vi "Main.vi"() -> ()   [LabVIEW 2019]
uses:
  main_control.ctl
  invader.ctl
  <vilib>/picture/picture.llb/imagedata.ctl
  move_dir_lr.ctl
  <vilib>/Utility/miscctls.llb/LVBoundsTypeDef.ctl
  shot_direction.ctl
  <vilib>/numeric/Random Number (Range) U64.vi
  <vilib>/numeric/Random Number (Range) DBL.vi
  <vilib>/numeric/sub_Random U32.vi
  <vilib>/Utility/inputDevices.llb/keyboardAcquire.vi
panel:
  out "output cluster":cluster{"x":i16, "y":i16}
  out "ShotPos_OUT":T1(array[cluster])
  in  "shotwidth":i16=10
  in  "speed":i16=10
  in  "smoothness":u32=10
  out "game":picture
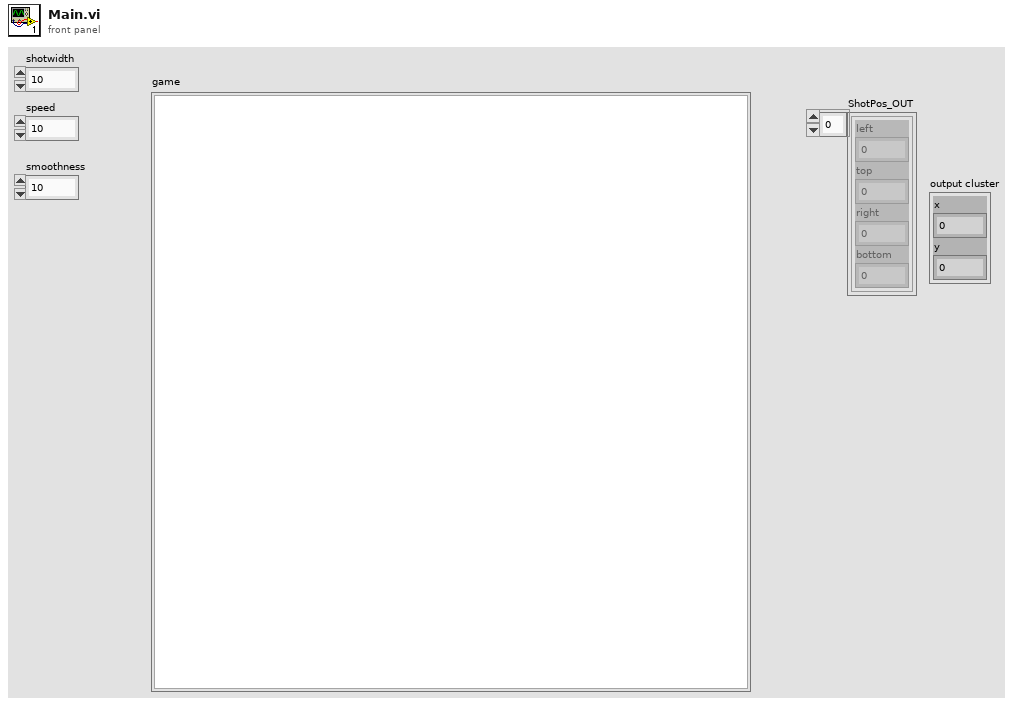
[diagram p1: front panel]
types:
  T1 = cluster{"left":i16, "top":i16, "right":i16, "bottom":i16}[]
  T2 = cluster{"left":i16, "top":i16, "right":i16, "bottom":i16}
  T3 = typedef "move_dir_lr.ctl" = enum16{"right", "left"}
  T4 = typedef "invader.ctl" = cluster{"output cluster":T5, "direction":T3, "shot_period":dbl, "Speed":i16, "Bounds":T6}
  T5 = typedef "imagedata.ctl" = cluster{"image type":i32, "image depth":i32, "image":u8[], "mask":u8[], "colors":u32[], "Rectangle":cluster{"left":i16, "top":i16, "right":i16, "bottom":i16}}
  T6 = typedef "LVBoundsTypeDef.ctl" = cluster{"Width":u32, "Height":u32}
  T7 = typedef "main_control.ctl" = enum16{"Idle", "RedrawPic"}
  T8 = typedef "shot_direction.ctl" = enum16{"down", "up"}
  T9 = cluster{"Font Name:":string, "Size":i16, "Strikeout?":bool, "Italic?":bool, "Underline?":bool, "Outline?":bool, "Shadow?":bool, "Bold?":bool}
  T10 = enum16{"User-specified Font", "Application Font", "System Font", "Dialog Font"}
  T11 = enum16{"0", "1", "2", "3", "4", "5", "6", "7", "8", "9", "A", "B", "C", "D", "E", "F", "G", "H", "I", "J", "K", "L", "M", "N", "O", "P", "Q", "R", "S", "T", "U", "V", "W", "X", "Y", "Z", "F1", "F2", "F3", "F4", "F5", "F6", "F7", "F8", "F9", "F10", "F11", "F12", "F13", "F14", "F15", "ADD", "BACK", "BACKSLASH", "CAPITAL", "COMMA", "DECIMAL", "DELETE", "DIVIDE", "DOWN", "END", "EQUALS", "ESCAPE", "GRAVE (`)", "HOME", "INSERT", "LBRACKET", "LCONTROL", "LEFT", "L ALT", "LSHIFT", "LWIN", "MINUS", "MULTIPLY", "NEXT", "NUMLOCK", "NUMPAD_0", "NUMPAD_1", "NUMPAD_2", "NUMPAD_3", "NUMPAD_4", "NUMPAD_5", "NUMPAD_6", "NUMPAD_7", "NUMPAD_8", "NUMPAD_9", "PAUSE", "PERIOD", "PRIOR (PG UP)", "RBRACKET", "RCONTROL", "RETURN", "RIGHT", "R ALT", "RSHIFT", "RWIN", "SCROLL", "SEMICOLON", "SLASH", "SPACE", "SUBTRACT", "TAB", "UP", "ENTER (num pad)", "' (quote)"}[]
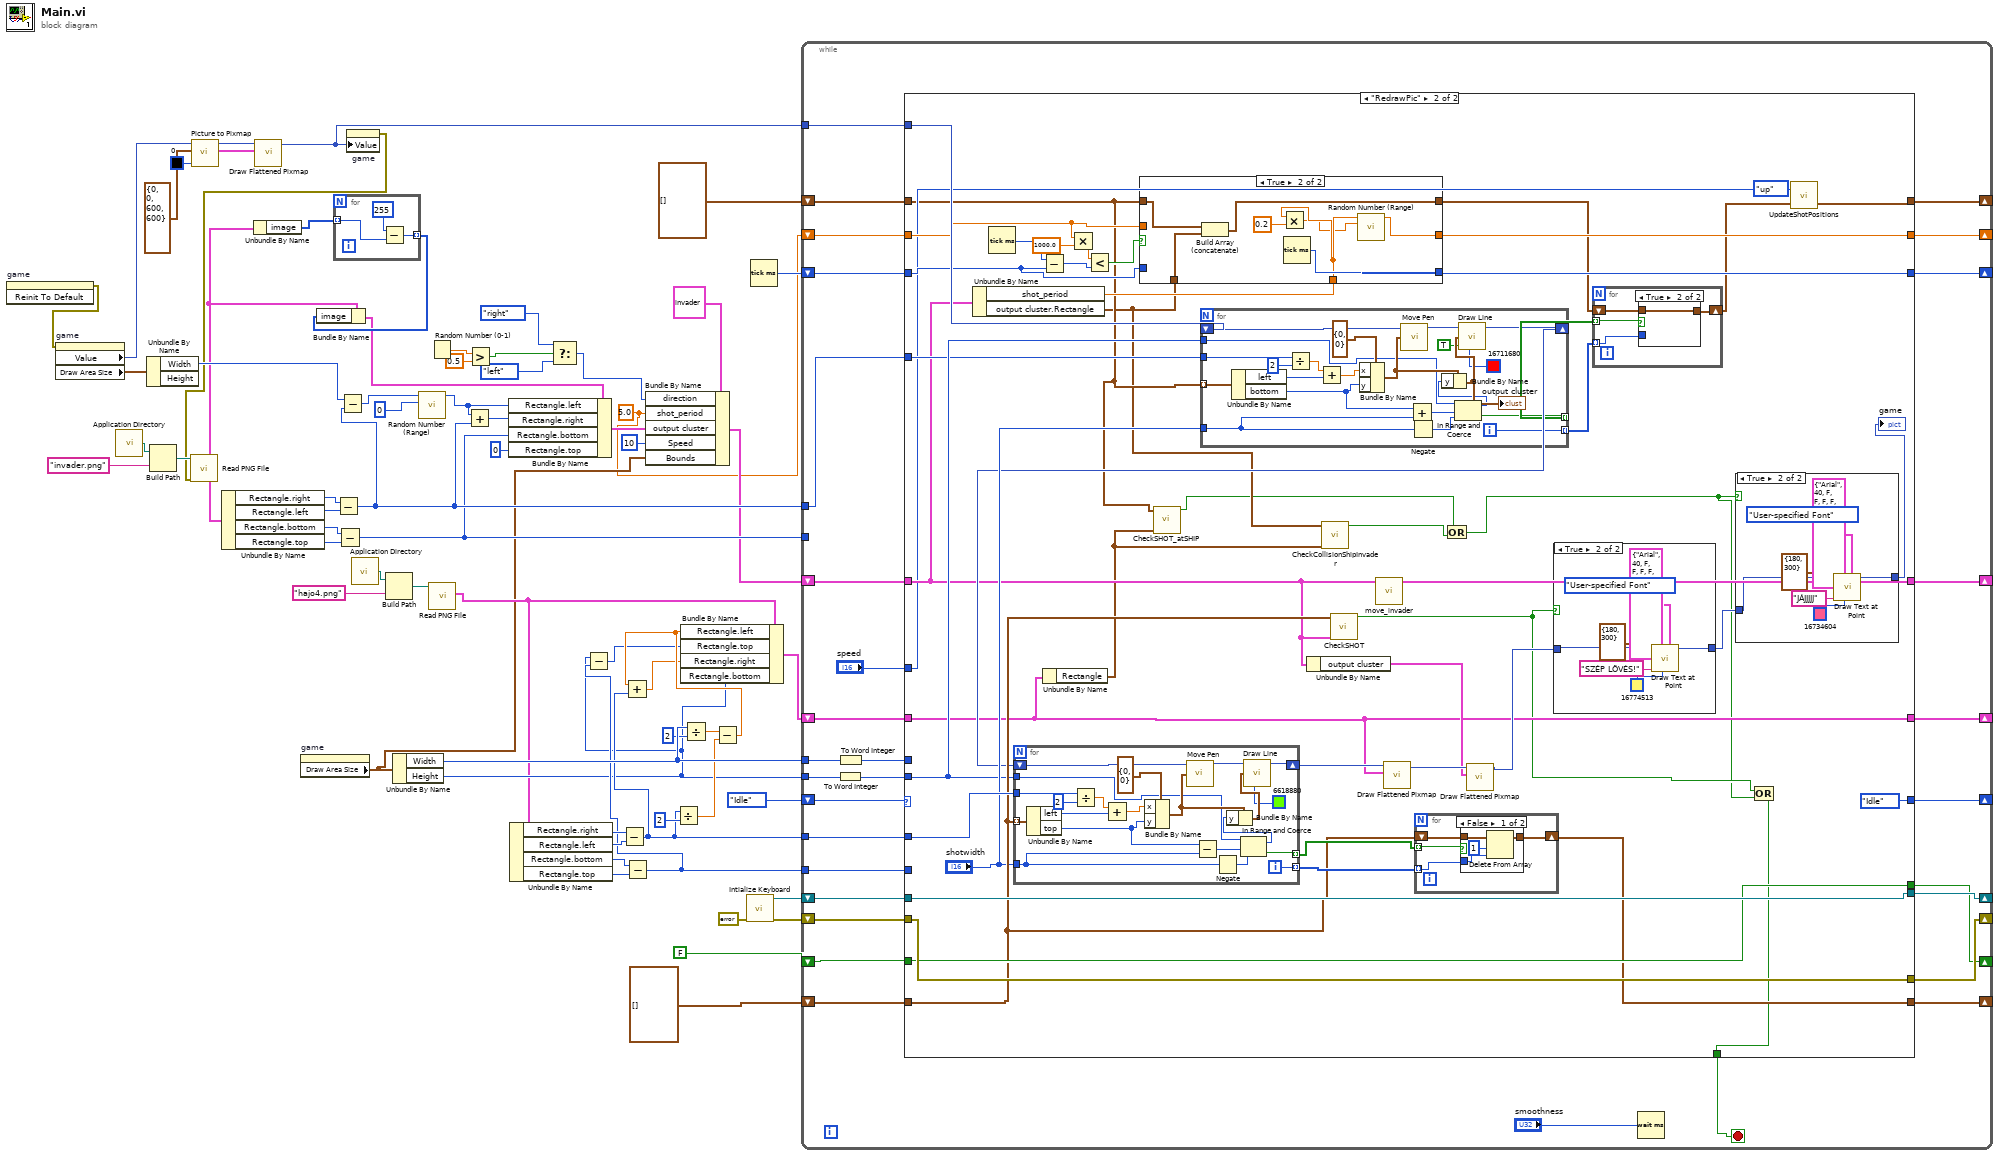
[diagram p0: block diagram]
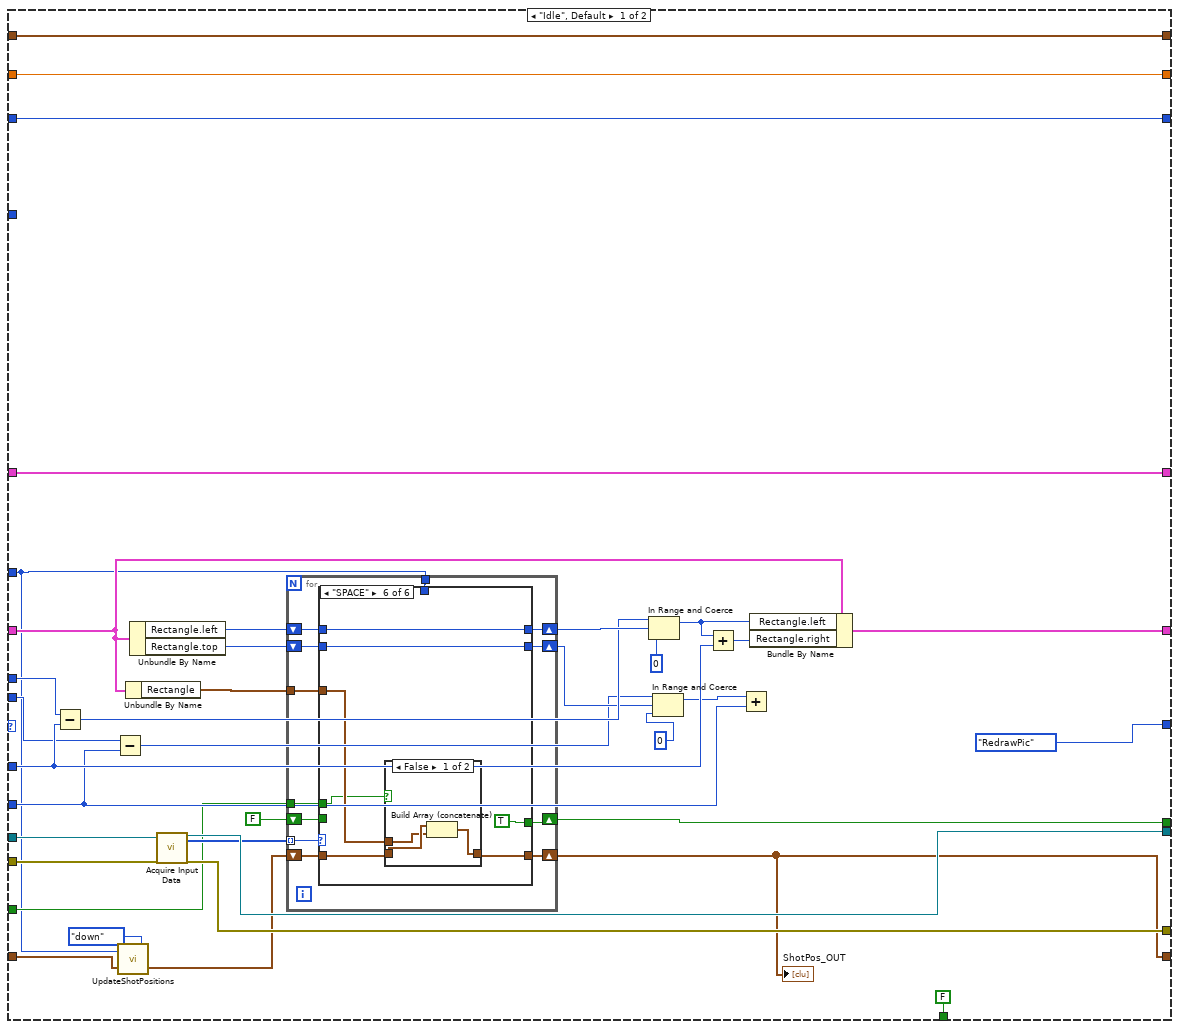
[diagram p2: hidden frame]
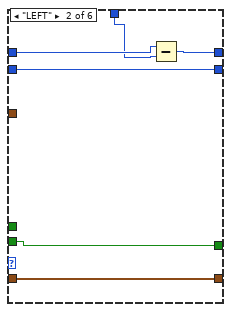
[diagram p4: hidden frame]
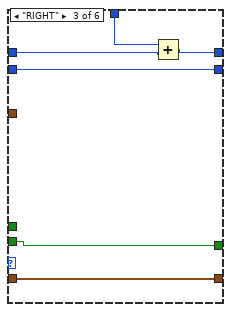
[diagram p5: hidden frame]
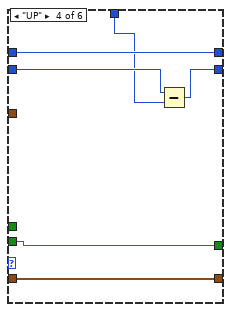
[diagram p6: hidden frame]
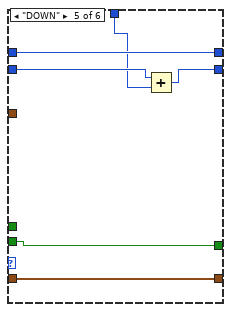
[diagram p7: hidden frame]
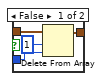
[diagram p10: hidden frame]
diagram:
  w1 = 5.0 ("shot_period")
  n1 = invoke on="game" class="Pict" method="Reinit To Default"() -> (error out=w4:errorcluster)  [unwired: 3 in, 2 out]
  n2 = property on="game" class="Pict"(error in=w4) -> ("Value"=w11:picture, "Draw Area Size"=w35:T6)  [unwired: 1 in, 2 out]
  n3 = call <vilib>:"Application Directory.vi"() -> ("Application Directory"=w41:path)
  n4 = Unbundle By Name(w35) -> ("Width"=w34:u32)  [unwired: 1 out]
  n5 = Build Path(base path=w41, name or relative path="invader.png") -> (appended path=w43:path)
  n6 = call <vilib>:"Picture to Pixmap.vi"("Background Color"=u32 0, "rect"=T2 {"left"=0, "top"=0, "right"=600, "bottom"=600}, "picture"=w11) -> ("image data"=w7:T5, "new picture"=w8:picture)  [unwired: 7 in]
  n7 = call <vilib>:"Draw Flattened Pixmap.vi"("image data"=w7, "picture"=w8) -> ("new picture"=w5:picture)  [unwired: 7 in]
  n8 = property on="game" class="Pict"() -> ("Draw Area Size"=w16:T6)  [unwired: 2 in, 2 out]
  n9 = property on="game" class="Pict"("Value"=w5) -> (error out=w6:errorcluster)  [unwired: 2 in, 1 out]
  n10 = call <vilib>:"Read PNG File.vi"("error in (no error)"=w6, "path to PNG file"=w43) -> ("image data"=w14:T5)  [unwired: 7 in, 2 out]
  n11 = Unbundle By Name(w14) -> ("Rectangle.right"=w40:i16, "Rectangle.left"=w39:i16, "Rectangle.bottom"=w38:i16, "Rectangle.top"=w37:i16)
  n12 = Unbundle By Name(w14) -> ("image"=w15:u8[])
  n13 = for {
    tunnel: w15 -> [w70] mode=indexing
    tunnel: [w69] -> w13 mode=indexing
    n14 = Subtract(x=u8 255, y=w70) -> (x-y=w69:u8)
  }
  n15 = Bundle By Name(cluster=w14, "image"=w13) -> (w12:T5)
  n16 = Subtract(x=w40, y=w39) -> (x-y=w31:i16)
  n17 = Subtract(x=w38, y=w37) -> (x-y=w28:i16)
  n18 = Subtract(x=w34, y=w31) -> (x-y=w33:u32)
  n19 = call <vilib>:"Application Directory.vi"() -> ("Application Directory"=w68:path)
  n20 = Build Path(base path=w68, name or relative path="hajo4.png") -> (appended path=w66:path)
  n21 = Unbundle By Name(w16) -> ("Width"=w55:u32, "Height"=w45:u32)
  n22 = call-poly <vilib>:"Random Number (Range).vi"("lower bound (0)"=u64 0, "upper bound (100)"=w33) -> ("number"=w32:u64)  [unwired: 9 in]
  n23 = Random Number (0-1)() -> (number: 0 to 1=w24:dbl)
  n24 = call <vilib>:"Read PNG File.vi"("path to PNG file"=w66) -> ("image data"=w18:T5)  [unwired: 8 in, 2 out]
  n25 = Add(x=w32, y=w31) -> (x+y=w30:u64)
  n26 = Greater?(x=w24, y=0.5) -> (0:w22:bool)
  n27 = Bundle By Name(cluster=w12, "Rectangle.left"=w32, "Rectangle.right"=w30, "Rectangle.bottom"=w28, "Rectangle.top"=i16 0) -> (w25:T5)
  n28 = Unbundle By Name(w18) -> ("Rectangle.right"=w65:i16, "Rectangle.left"=w64:i16, "Rectangle.bottom"=w63:i16, "Rectangle.top"=w62:i16)
  n29 = Select(t=move_dir_lr."right" ("direction"), s=w22, f=move_dir_lr."left" ("direction")) -> (s? t:f=w19:T3)
  n30 = Subtract(x=w65, y=w64) -> (x-y=w49:i16)
  n31 = Subtract(x=w63, y=w62) -> (x-y=w47:i16)
  n32 = Subtract(x=w45, y=w47) -> (x-y=w46:u32)
  n33 = Bundle By Name(cluster=T4 {"output cluster"={"image type"=0, "image depth"=0, "image"=[], "mask"=[], "colors"=[], "Rectangle"={"left"=0, "top"=0, "right"=0, "bottom"=0}}, "direction"=enum."right", "shot_period"=0.0, "Speed"=10, "Bounds"={"Width"=0, "Height"=0}} ("input cluster"), "direction"=w19, "shot_period"=w1, "output cluster"=w25, "Speed"=i16 10, "Bounds"=w16) -> (w26:T4)
  n34 = Divide(x=w49, y=u32 2) -> (x/y=w51:dbl)
  n35 = Divide(x=w55, y=u32 2) -> (x/y=w53:dbl)
  n36 = Subtract(x=w53, y=w51) -> (x-y=w50:dbl)
  n37 = Add(x=w50, y=w49) -> (x+y=w48:dbl)
  n38 = Bundle By Name(cluster=w18, "Rectangle.left"=w50, "Rectangle.top"=w46, "Rectangle.right"=w48, "Rectangle.bottom"=w45) -> (w44:T5)
  n39 = call <vilib>:"Intialize Keyboard.vi"("error in (no error)"=errorcluster {"status"=FALSE, "code"=0, "source"=""}) -> ("error out"=w59:errorcluster, "device ID"=w60:refnum<k1>)  [unwired: 9 in]
  n40 = Tick Count (ms)() -> (millisecond timer value=w2:u32)
  n41 = while {
    tunnel: w49 -> [w102]
    tunnel: w55 -> [w93]
    tunnel: w47 -> [w99]
    tunnel: w45 -> [w88]
    shift-right: [w96] -> _
    shift-left: main_control."Idle" -> [w98]
    shift-right: [w97] -> _
    shift-left: w44 -> [w101]
    shift-right: [w90] -> _
    shift-left: w60 -> [w95]
    shift-right: [w89] -> _
    shift-left: w59 -> [w94]
    shift-right: [w85] -> _
    shift-left: T1 [] -> [w86]
    shift-right: [w83] -> _
    shift-left: FALSE -> [w84]
    tunnel: w31 -> [w76]
    tunnel: w28 -> [_]
    shift-right: [w81] -> _
    shift-left: w26 -> [w82]
    tunnel: w5 -> [w80]
    shift-right: [w78] -> _
    shift-left: T1 [] -> [w79]
    shift-right: [w75] -> _
    shift-left: w2 -> [w77]
    shift-right: [w73] -> _
    shift-left: w1 -> [w74]
    stop <- w91 stop-if-true
    n42 = To Word Integer(number=w88) -> (16bit integer=w87:i16)
    n43 = To Word Integer(number=w93) -> (16bit integer=w92:i16)
    n44 = case shown="\"RedrawPic\"" w98 {
      tunnel: w101 -> [w118 w200]
      tunnel: [w135 w200] -> w97
      tunnel: [main_control."RedrawPic" main_control."Idle"] -> w96
      tunnel: w102 -> [w136 w234]
      tunnel: w99 -> [w120 _]
      tunnel: w92 -> [w137 _]
      tunnel: w87 -> [w125 w222]
      tunnel: w95 -> [w139 w237]
      tunnel: w94 -> [w138 w236]
      tunnel: [FALSE ("SHOT") w196] -> w91
      tunnel: [w134 w237] -> w90
      tunnel: [w133 w236] -> w89
      tunnel: w86 -> [w114 w226]
      tunnel: [w115 w227] -> w85
      tunnel: w84 -> [w112 w231]
      tunnel: [w110 w231] -> w83
      tunnel: w82 -> [w109 w220]
      tunnel: [w109 w228] -> w81
      tunnel: w80 -> [_ w224]
      tunnel: w79 -> [w107 w201]
      tunnel: [w107 w204] -> w78
      tunnel: w77 -> [w105 w215]
      tunnel: w76 -> [_ w221]
      tunnel: [w105 w216] -> w75
      tunnel: w74 -> [w106 w209]
      tunnel: [w106 w214] -> w73
      tunnel: "speed" -> [w104 w206]
      frame "Idle", Default {
        n45 = Subtract(x=w137, y=w136) -> (x-y=w128:i16)
        n46 = Subtract(x=w125, y=w120) -> (x-y=w121:i16)
        n47 = call "UpdateShotPositions.vi"("Direction"=shot_direction."down", "ShotPos_IN"=w114, "Speed"=w104) -> ("ShotPos_OUT"=w116:T1)
        n48 = Unbundle By Name(w118) -> ("Rectangle"=w117:T2)
        n49 = Unbundle By Name(w118) -> ("Rectangle.left"=w131:i16, "Rectangle.top"=w124:i16)
        n50 = call-poly <vilib>:"Acquire Input Data.vi"("device ID"=w139, "error in (no error)"=w138) -> ("device ID"=w134:refnum<k1>, "keys pressed"=w132:T11, "error out"=w133:errorcluster)  [unwired: 15 in]
        n51 = for {
          tunnel: w132 -> [w151] mode=indexing
          shift-right: [w150] -> w130
          shift-left: w131 -> [w149]
          shift-right: [w147] -> w122
          shift-left: w124 -> [w148]
          tunnel: w104 -> [w146]
          tunnel: w117 -> [w145]
          shift-right: [w143] -> w115
          shift-left: w116 -> [w144]
          shift-right: [w141] -> w110
          shift-left: FALSE -> [w142]
          tunnel: w112 -> [w140]
          n52 = case shown="\"SPACE\"" w151 {
            tunnel: w149 -> [w155 w160 w166 w173 w179 w186]
            tunnel: [w155 w158 w165 w173 w179 w186] -> w150
            tunnel: w148 -> [w154 w161 w167 w172 w178 w185]
            tunnel: [w154 w161 w167 w170 w176 w185] -> w147
            tunnel: w146 -> [_ w159 w164 w171 w177 _]
            tunnel: w145 -> [_ _ _ _ _ w183]
            tunnel: w144 -> [w153 w157 w163 w169 w175 w184]
            tunnel: [w153 w157 w163 w169 w175 w182] -> w143
            tunnel: w142 -> [w152 w156 w162 w168 w174 _]
            tunnel: [w152 w156 w162 w168 w174 TRUE] -> w141
            tunnel: w140 -> [_ _ _ _ _ w181]
            frame Default {
            }
            frame "LEFT" {
              n53 = Subtract(x=w160, y=w159) -> (x-y=w158:i16)
            }
            frame "RIGHT" {
              n54 = Add(x=w164, y=w166) -> (x+y=w165:i16)
            }
            frame "UP" {
              n55 = Subtract(x=w172, y=w171) -> (x-y=w170:i16)
            }
            frame "DOWN" {
              n56 = Add(x=w178, y=w177) -> (x+y=w176:i16)
            }
            frame "SPACE" {
              n57 = case shown="False" w181 {
                tunnel: w184 -> [w189 w190]
                tunnel: w183 -> [w188 _]
                tunnel: [w187 w190] -> w182
                frame False {
                  n58 = Build Array (concatenate)(w189, w188) -> (w187:T1)
                }
                frame True {
                }
              }
            }
          }
        }
        "ShotPos_OUT" <- w115
        n59 = In Range and Coerce(upper limit=w128, x=w130, lower limit=i16 0) -> (coerced(x)=w127:i16)  [unwired: 1 out]
        n60 = In Range and Coerce(upper limit=w121, x=w122, lower limit=i16 0) -> (coerced(x)=w119:i16)  [unwired: 1 out]
        n61 = Add(x=w127, y=w136) -> (x+y=w126:i16)
        n62 = Add(x=w119, y=w120) -> ()  [unwired: 1 out]
        n63 = Bundle By Name(cluster=w118, "Rectangle.left"=w127, "Rectangle.right"=w126) -> (w135:T5)
      }
      frame "RedrawPic" {
        n64 = Unbundle By Name(w220) -> ("shot_period"=w213:dbl, "output cluster.Rectangle"=w195:T2)
        n65 = Tick Count (ms)() -> (millisecond timer value=w219:u32)
        n66 = Subtract(x=w219, y=w215) -> (x-y=w218:u32)
        n67 = Unbundle By Name(w200) -> ("Rectangle"=w194:T2)
        n68 = Multiply(x=w209, y=1000.0) -> (x*y=w207:dbl)
        n69 = Less?(x=w207, y=w218) -> (x < y?=w217:bool)
        n70 = case shown="True" w217 {
          tunnel: w201 -> [w258 w266]
          tunnel: w195 -> [_ w265]
          tunnel: [w258 w264] -> w210
          tunnel: [w257 w263] -> w216
          tunnel: w215 -> [w257 _]
          tunnel: [w256 w259] -> w214
          tunnel: w213 -> [_ w262]
          tunnel: w209 -> [w256 _]
          frame False {
          }
          frame True {
            n71 = Build Array (concatenate)(w266, w265) -> (w264:T1)
            n72 = Multiply(x=w262, y=0.2) -> (x*y=w260:dbl)
            n73 = Tick Count (ms)() -> (millisecond timer value=w263:u32)
            n74 = call-poly <vilib>:"Random Number (Range).vi"("lower bound (0)"=w260, "upper bound (100)"=w262) -> ("number"=w259:dbl)  [unwired: 9 in]
          }
        }
        n75 = call "CheckSHOT_atSHIP.vi"("ShipRectangle"=w194, "InvaderShotArray"=w201) -> ("SHOT"=w192:bool)  [unwired: 9 in]
        n76 = for {
          tunnel: w201 -> [w287] mode=indexing
          shift-right: [w275] -> w223
          shift-left: w224 -> [w288]
          tunnel: w221 -> [w286]
          tunnel: [w274] -> w212 mode=indexing
          tunnel: w222 -> [w268]
          tunnel: [w271] -> w211 mode=indexing
          tunnel: "shotwidth" -> [w269]
          i -> [w271]
          n77 = Unbundle By Name(w287) -> ("left"=w283:i16, "bottom"=w278:i16)
          n78 = Divide(x=w286, y=i16 2) -> (x/y=w284:dbl)
          n79 = Add(x=w284, y=w283) -> (x+y=w282:dbl)
          n80 = Bundle By Name(cluster=cluster{"x":i16, "y":i16} {"x"=0, "y"=0} ("new position"), "x"=w282, "y"=w278) -> (w279:cluster{"x":i16, "y":i16})
          n81 = call <vilib>:"Move Pen.vi"("new position"=w279, "picture"=w288) -> ("new picture"=w281:picture)  [unwired: 3 in]
          n82 = Add(x=w278, y=w269) -> (x+y=w273:i16)
          n83 = Negate(x=w269) -> (-x=w267:i16)
          n84 = In Range and Coerce(upper limit=w268, x=w273, lower limit=w267) -> (coerced(x)=w272:i16, In Range?=w274:bool)
          n85 = Bundle By Name(cluster=w279, "y"=w272) -> (w277:cluster{"x":i16, "y":i16})
          "output cluster" <- w277
          n86 = call <vilib>:"Draw Line.vi"("picture"=w281, "end point"=w277, "absolute coordinates?(T)"=TRUE, "color(black)"=u32 16711680) -> ("new picture"=w275:picture)  [unwired: 5 in]
        }
        n87 = for {
          tunnel: w226 -> [w325] mode=indexing
          shift-right: [w314] -> w235
          shift-left: w223 -> [w326]
          tunnel: w234 -> [w324]
          tunnel: [w313] -> w232 mode=indexing
          tunnel: w222 -> [w310]
          tunnel: [w308] -> w233 mode=indexing
          tunnel: "shotwidth" -> [w306]
          i -> [w308]
          n88 = Unbundle By Name(w325) -> ("left"=w321:i16, "top"=w316:i16)
          n89 = Divide(x=w324, y=i16 2) -> (x/y=w322:dbl)
          n90 = Add(x=w322, y=w321) -> (x+y=w320:dbl)
          n91 = Bundle By Name(cluster=cluster{"x":i16, "y":i16} {"x"=0, "y"=0} ("new position"), "x"=w320, "y"=w316) -> (w317:cluster{"x":i16, "y":i16})
          n92 = call <vilib>:"Move Pen.vi"("new position"=w317, "picture"=w326) -> ("new picture"=w319:picture)  [unwired: 3 in]
          n93 = Subtract(x=w316, y=w306) -> (x-y=w312:i16)
          n94 = Negate(x=w306) -> (-x=w311:i16)
          n95 = In Range and Coerce(upper limit=w310, x=w312, lower limit=w311) -> (coerced(x)=w309:i16, In Range?=w313:bool)
          n96 = Bundle By Name(cluster=w317, "y"=w309) -> (w315:cluster{"x":i16, "y":i16})
          n97 = call <vilib>:"Draw Line.vi"("picture"=w319, "end point"=w315, "color(black)"=u32 6618880) -> ("new picture"=w314:picture)  [unwired: 6 in]
        }
        n98 = Unbundle By Name(w220) -> ("output cluster"=w229:T5)
        n99 = call "CheckCollisionShipInvader.vi"("ShipRectangle"=w194, "InvaderRectangle"=w195) -> ("Collision"=w193:bool)  [unwired: 9 in]
        n100 = call "CheckSHOT.vi"("invader_in"=w220, "Array"=w226) -> ("SHOT"=w197:bool)  [unwired: 9 in]
        n101 = call "move_invader.vi"("invader_in"=w220) -> ("invader_out"=w228:T4)  [unwired: 10 in]
        n102 = call <vilib>:"Draw Flattened Pixmap.vi"("image data"=w200, "picture"=w235) -> ("new picture"=w230:picture)  [unwired: 7 in]
        n103 = for {
          tunnel: w232 -> [w298] mode=indexing
          tunnel: w233 -> [w297] mode=indexing
          shift-right: [w299] -> w227
          shift-left: w226 -> [w300]
          n104 = case shown="False" w298 {
            tunnel: w300 -> [w304 w305]
            tunnel: [w303 w305] -> w299
            tunnel: w297 -> [w302 _]
            frame False {
              n105 = Delete From Array(array=w304, length=1, index=w302) -> (array with subset deleted=w303:T1)  [unwired: 1 out]
            }
            frame True {
            }
          }
        }
        n106 = Or(x=w192, y=w193) -> (x .or. y?=w191:bool)
        n107 = call <vilib>:"Draw Flattened Pixmap.vi"("image data"=w229, "picture"=w230) -> ("new picture"=w202:picture)  [unwired: 7 in]
        n108 = case shown="True" w197 {
          tunnel: w202 -> [w289 w293]
          tunnel: [w289 w296] -> w199
          frame False {
          }
          frame True {
            n109 = call <vilib>:"Draw Text at Point.vi"("[user-specified font]"=T9 {"Font Name:"="Arial", "Size"=40, "Strikeout?"=FALSE, "Italic?"=FALSE, "Underline?"=FALSE, "Outline?"=FALSE, "Shadow?"=FALSE, "Bold?"=FALSE}, "text color(black)"=u32 16774513, "desired font(Application)"=T10."User-specified Font", "text"="SZÉP LÖVÉS!", "origin"=cluster{"x":i16, "y":i16} {"x"=180, "y"=300}, "picture"=w293) -> ("new picture"=w296:picture)  [unwired: 4 in, 1 out]
          }
        }
        n110 = for {
          tunnel: w212 -> [w248] mode=indexing
          tunnel: w211 -> [w247] mode=indexing
          shift-right: [w249] -> w205
          shift-left: w210 -> [w250]
          n111 = case shown="True" w248 {
            tunnel: w250 -> [w254 w255]
            tunnel: [w253 w255] -> w249
            tunnel: w247 -> [w252 _]
            frame False {
              n112 = Delete From Array(array=w254, length=1, index=w252) -> (array with subset deleted=w253:T1)  [unwired: 1 out]
            }
            frame True {
            }
          }
        }
        n113 = case shown="True" w191 {
          tunnel: w199 -> [w239 w243]
          tunnel: [w239 w246] -> w198
          frame False {
          }
          frame True {
            n114 = call <vilib>:"Draw Text at Point.vi"("[user-specified font]"=T9 {"Font Name:"="Arial", "Size"=40, "Strikeout?"=FALSE, "Italic?"=FALSE, "Underline?"=FALSE, "Outline?"=FALSE, "Shadow?"=FALSE, "Bold?"=FALSE}, "text color(black)"=u32 16734604, "desired font(Application)"=T10."User-specified Font", "text"="JÁJJJJJ", "origin"=cluster{"x":i16, "y":i16} {"x"=180, "y"=300}, "picture"=w243) -> ("new picture"=w246:picture)  [unwired: 4 in, 1 out]
          }
        }
        "game" <- w198
        n115 = Or(x=w197, y=w191) -> (x .or. y?=w196:bool)
        n116 = call "UpdateShotPositions.vi"("Direction"=shot_direction."up", "ShotPos_IN"=w205, "Speed"=w206) -> ("ShotPos_OUT"=w204:T1)
      }
    }
    n117 = Wait (ms)(milliseconds to wait="smoothness") -> ()  [unwired: 1 out]
  }
